vi "Create from Listener.vi"(8 "Error In":errorcluster, 11 "Listener":refnum<class "Listener.lvclass">) -> (0 "Error Out":errorcluster, 3 "Channel":refnum<class "Channel.lvclass">)   [LabVIEW 2018, in "Toolkit.lvlib" / "Channel.lvclass"]
uses:
  Channel.lvclass
  Listener/Listener.lvclass
  Listener/Listener.lvclass/Listener.ctl
  Session/Session.lvclass/Session.ctl
  SSH/SSH.lvclass/SSH.ctl
  Channel.lvclass/Channel.ctl
  Session/Session.lvclass
  Toolkit.lvlib
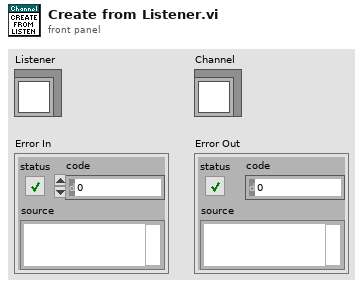
[diagram p1: front panel]
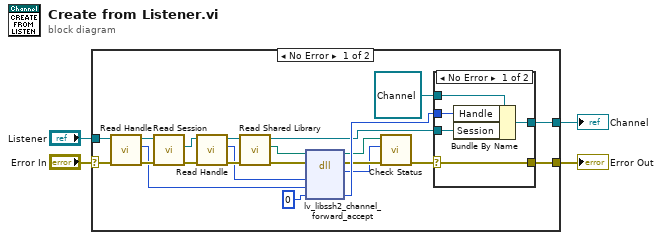
[diagram p0: block diagram]
diagram:
  n1 = case shown="No Error" "Error In" {
    selector: "Error In" -> [w10 w34]
    tunnel: [w14 w34] -> w3
    tunnel: [w26 _] -> w2
    tunnel: "Listener" -> [w11 _]
    frame No Error {
      n2 = call "Read Handle.vi"("Error In"=w10, "Listener In"=w11) -> ("Error Out"=w8:errorcluster, "Handle"=w5:u64, "Listener Out"=w9:refnum<class "Listener.lvclass">)  [unwired: 7 in]
      n3 = call "Read Session.vi"("Error In"=w8, "Listener In"=w9) -> ("Error Out"=w6:errorcluster, "Session"=w7:refnum<class "Session.lvclass">)  [unwired: 7 in, 1 out]
      n4 = call "Read Handle.vi"("Error In"=w6, "Session In"=w7) -> ("Erorr Out"=w24:errorcluster, "Handle"=w21:u64, "Session Out"=w25:refnum<class "Session.lvclass">)  [unwired: 7 in]
      n5 = call "Read Shared Library.vi"("Error In"=w24, "Session In"=w25) -> ("Erorr Out"=w23:errorcluster, "libssh2lv Shared Library"=w22:path, "Session Out"=w13:refnum<class "Session.lvclass">)  [unwired: 7 in]
      n6 = dll-call lib="libssh2lv.*" fn="lv_libssh2_channel_forward_accept"(path in=w22, error in=w23, "session"=w21, "listener"=w5, "handle"=u64 0) -> (path out=w16:path, error out=w18:errorcluster, "status"=w17:i32, "handle"=w19:u64)  [unwired: 3 in]
      n7 = call "Check Status.vi"("Error In"=w18, "Status"=w17, "lv-libssh2 Shared Library In"=w16) -> ("Error Out"=w15:errorcluster)  [unwired: 7 in, 1 out]
      n8 = case shown="No Error" w15 {
        selector: w15 -> [w30 w33]
        tunnel: [w27 w32] -> w26
        tunnel: w19 -> [w31 _]
        tunnel: [w30 w33] -> w14
        tunnel: w13 -> [w29 _]
        tunnel: refnum<class "Channel.lvclass"> refnum ("Toolkit.lvlib:Channel.lvclass") -> [w28 w32]
        frame No Error {
          n9 = Bundle By Name(cluster=w28, "Handle"=w31, "Session"=w29) -> (w27:refnum<class "Channel.lvclass">)
        }
        frame Error {
        }
      }
    }
    frame Error {
    }
  }
  "Error Out" <- w3
  "Channel" <- w2
